vi "ToRepo.vi"(8 "error in":errorcluster, 9 "to repo cluster":T1, 10 "repository in":refnum<class "NISE_CEF_Repository.lvclass">, 11 "node in":refnum<class "Initialization.lvclass">) -> (0 "error out":errorcluster, 2 "repository out":refnum<class "NISE_CEF_Repository.lvclass">, 3 "node out":refnum<class "Initialization.lvclass">)   [LabVIEW 2019, in "Initialization.lvclass"]
doc: "Transfers the information from the tree node into the repo. How it is stored in the repo depends on the Repo.Copyright 2015 National Instruments Corporation\n\nLicensed under the Apache License, Version 2.0 (the \"License\"); you may not use this file except in compliance with the License. You may obtain a copy of the License at http://www.apache.org/licenses/LICENSE-2.0\nUnless required by applicable law or agreed to in writing, software distributed under the License is distributed on an \"AS IS\" BASIS, WITHOUT WARRANTIES OR CONDITIONS OF ANY KIND, either express or implied. See the License for the specific language governing permissions and limitations under the License."
uses:
  Initialization.lvclass
  <vilib>/NI/Configuration Framework/Repository/NISE_CEF_Repository.lvclass
  <vilib>/NI/Configuration Framework/Node/ToRepoCluster.ctl
  CustomDeviceRepo/CustomDeviceRepo.lvclass
  C:/Program Files (x86)/National Instruments/LabVIEW 2019/vi.lib/NI/Configuration Framework/Repository/NISE_CEF_Repository.lvclass
  Initialization.lvclass/Initialization.ctl
  CustomDeviceRepo/CustomDeviceRepo.lvclass/CustomDeviceRepo.ctl
  CustomDeviceRepo/Write Initialization VI Properties.vi
  <vilib>/NI/Configuration Framework/Node/NISE_CEF_Node.lvclass
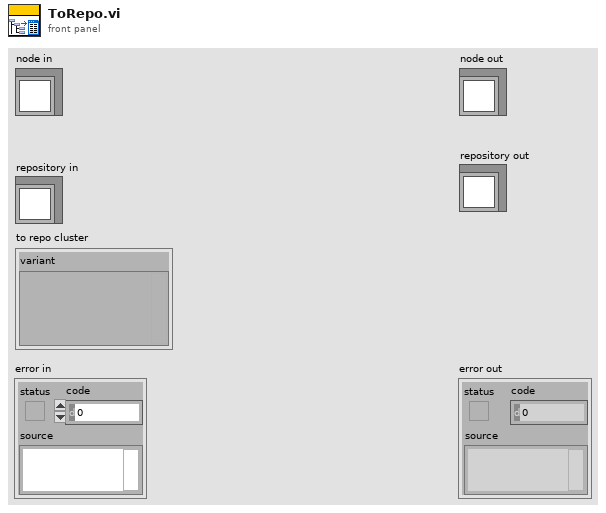
[diagram p1: front panel]
types:
  T1 = typedef "NISE_CEF_Node.lvclass/ToRepoCluster.ctl" = cluster{"variant":variant}
  T2 = typedef "VeriStand Custom Device XML Parser.lvlib/Initialization VI Properties.ctl" = cluster{"Execution":T3, "Path":T4, "Type":enum16{"Action", "VI"}, "Position":enum16{"centered", "mouse pointer"}}
  T3 = typedef "VeriStand Custom Device XML Parser.lvlib/Execution Types.ctl" = enum16{"silent", "modal", "floating", "default"}
  T4 = typedef "VeriStand Custom Device XML Parser.lvlib/Path Cluster.ctl" = cluster{"Path":path, "Path Type":enum16{"Absolute", "To Base", "To Common Doc Dir", "To Application Data Dir"}}
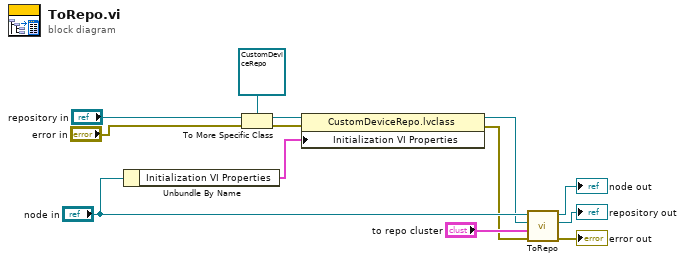
[diagram p0: block diagram]
diagram:
  n1 = Unbundle By Name("node in") -> ("Initialization VI Properties"=w4:T2)
  n2 = To More Specific Class(target class=refnum<class "CustomDeviceRepo.lvclass"> refnum ("CustomDeviceRepo.lvclass"), reference="repository in", error in="error in") -> (specific class reference=w8:refnum<class "CustomDeviceRepo.lvclass">, error out=w7:errorcluster)
  n3 = property class="CustomDeviceRepo.lvclass"(reference=w8, error in=w7, "Initialization VI Properties"=w4) -> (reference out=w2:refnum<class "CustomDeviceRepo.lvclass">, error out=w1:errorcluster)
  n4 = call-parent "ToRepo.vi"("error in"=w1, "to repo cluster"="to repo cluster", "repository in"=w2, "node in"="node in") -> ("error out"=→"error out":errorcluster, "repository out"=→"repository out":refnum<class "NISE_CEF_Repository.lvclass">, "node out"=→"node out":refnum<class "Initialization.lvclass">)  [unwired: 5 in]
